vi "Get Result.vi"(8 "error in (no error)":errorcluster, 11 "Channel Scanner in":refnum<class "Channel Scanner.lvclass">) -> (0 "error out":errorcluster, 2 "Result":refnum<class "Acquired Result.lvclass">, 3 "Channel Scanner out":refnum<class "Channel Scanner.lvclass">)   [LabVIEW 2015, in "Channel Scanner.lvclass"]
uses:
  Channel Scanner.lvclass
  Measure_core/Results/Acquired Result/Acquired Result.lvclass
  Channel Scanner.lvclass/Channel Scanner.ctl
  Read Channel scanner configuration.vi
  Measure_core/Instrument Recorders/Instrument Recorder/Instrument Recorder.lvclass
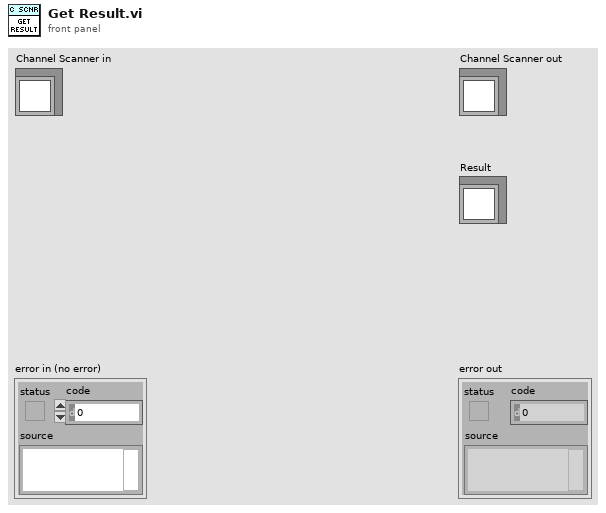
[diagram p1: front panel]
types:
  T1 = typedef "Channel Scanner Configuration.ctl" = cluster{"Scan channels":i32[], "Group with measurement":string}
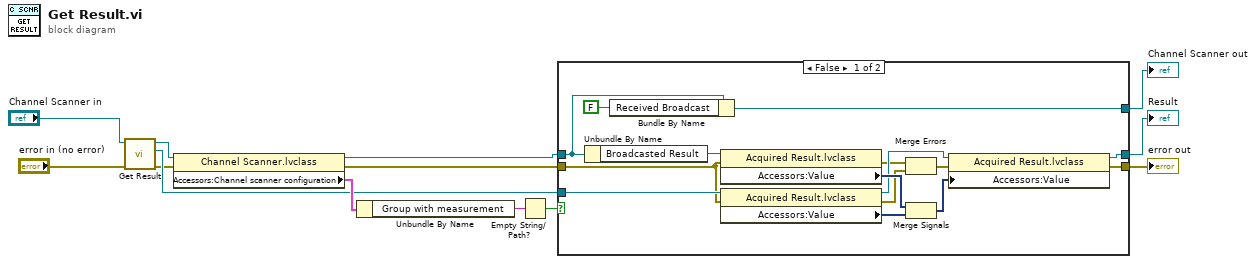
[diagram p0: block diagram]
diagram:
  n1 = call-parent "Get Result.vi"("error in (no error)"="error in (no error)", "Instrument Recorder in"="Channel Scanner in") -> ("error out"=w2:errorcluster, "Result"=w7:refnum<class "Acquired Result.lvclass">, "Instrument Recorder out"=w13:refnum<class "Channel Scanner.lvclass">)  [unwired: 7 in]
  n2 = property class="Channel Scanner.lvclass"(reference=w13, error in=w2) -> (reference out=w6:refnum<class "Channel Scanner.lvclass">, error out=w5:errorcluster, "Accessors:Channel scanner configuration"=w10:T1)
  n3 = Unbundle By Name(w10) -> ("Group with measurement"=w9:string)
  n4 = Empty String/Path?(string/path=w9) -> (empty?=w8:bool)
  n5 = case shown="False" w8 {
    tunnel: w7 -> [w26 w31]
    tunnel: w6 -> [w18 w30]
    tunnel: w5 -> [w23 w29]
    tunnel: [w19 w31] -> w4
    tunnel: [w17 w30] -> w3
    tunnel: [w15 w29] -> w1
    frame False {
      n6 = Unbundle By Name(w18) -> ("Broadcasted Result"=w28:refnum<class "Acquired Result.lvclass">)
      n7 = Bundle By Name(cluster=w18, "Received Broadcast"=FALSE) -> (w17:refnum<class "Channel Scanner.lvclass">)
      n8 = property class="Acquired Result.lvclass"(reference=w28, error in=w23) -> (error out=w24:errorcluster, "Accessors:Value"=w27:dynamicdata)  [unwired: 1 out]
      n9 = property class="Acquired Result.lvclass"(reference=w26, error in=w23) -> (reference out=w25:refnum<class "Acquired Result.lvclass">, error out=w22:errorcluster, "Accessors:Value"=w20:dynamicdata)
      n10 = Merge Errors(w24, w22) -> (w21:errorcluster)
      n11 = Merge Signals(w27, w20) -> (w14:dynamicdata)
      n12 = property class="Acquired Result.lvclass"(reference=w25, error in=w21, "Accessors:Value"=w14) -> (reference out=w19:refnum<class "Acquired Result.lvclass">, error out=w15:errorcluster)
    }
    frame True {
    }
  }
  "error out" <- w1
  "Channel Scanner out" <- w3
  "Result" <- w4
